vi "RSZVB Query External Power Meter.vi"(8 "error in (no error)":errorcluster {"code" format="%.0x"}, 10 "Power Meter Number (1)":i32=1, 11 "VISA session":refnum<visa-resource-name>) -> (0 "error out":errorcluster {"code" format="%.0x"}, 1 "Power Meter Name":string, 3 "dup VISA session":refnum<visa-resource-name>, 4 "Interface Address":string, 5 "Interface Type":string, 7 "Power Meter Type":string)   [LabVIEW 2011]
doc: "This VI queries an external power meter.\n\nRemote-control command(s):\nSYSTem:COMMunicate:RDEVice:PMETer<pmeter_no>:DEFine?"
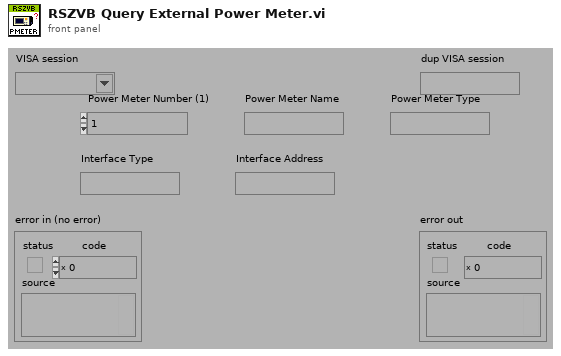
[diagram p1: front panel]
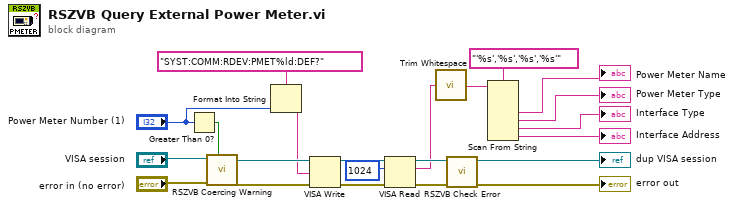
[diagram p0: block diagram]
diagram:
  n1 = Greater Than 0?(x="Power Meter Number (1)") -> (x > 0?=w9:bool)
  n2 = call "RSZVB Coercing Warning.vi"("In Range?"=w9, "error in (no error)"="error in (no error)", "VISA session"="VISA session") -> ("error out"=w13:errorcluster, "dup VISA session"=w12:refnum<visa-resource-name>)  [unwired: 7 in]
  n3 = Format Into String(format string="SYST:COMM:RDEV:PMET%ld:DEF?", "Power Meter Number (1)") -> (resulting string=w8:string)  [unwired: 2 in, 1 out]
  n4 = VISA Write(VISA resource name=w12, write buffer=w8, error in (no error)=w13) -> (VISA resource name out=w20:refnum<visa-resource-name>, error out=w22:errorcluster)  [unwired: 1 out]
  n5 = VISA Read(VISA resource name=w20, byte count=u32 1024 ("byte count (0)"), error in (no error)=w22) -> (VISA resource name out=w19:refnum<visa-resource-name>, read buffer=w17:string, error out=w18:errorcluster)  [unwired: 1 out]
  n6 = call <vilib>:"Trim Whitespace.vi"("string"=w17) -> ("trimmed string"=w5:string)  [unwired: 1 in]
  n7 = call "RSZVB Check Error.vi"("error in (no error)"=w18, "VISA session"=w19) -> ("error out"=→"error out":errorcluster, "dup VISA session"=→"dup VISA session":refnum<visa-resource-name>)  [unwired: 8 in]
  n8 = Scan From String(format string="'%s','%s','%s','%s'", input string=w5) -> (output 1=→"Power Meter Name":string, output 2=→"Power Meter Type":string, output 3=→"Interface Type":string, output 4=→"Interface Address":string)  [unwired: 6 in, 3 out]
